vi "Construct String Control Sink.vi"(4 "Error Action":T1=enum."Ignore Error and Close Sink", 5 "Buffer Length(0)":u32, 6 "Clear on Shutdown?(F)":bool, 7 "Str Refnum":refnum<vi>, 8 "Log Filter":refnum<class "ILogFilter.lvclass">, 9 "AutoScroll?(F)":bool, 10 "LogFormat":refnum<class "IStringFormat.lvclass">, 11 "LogLevel":T2) -> (3 "String Control Sink out":refnum<class "String Control Sink.lvclass">)   [LabVIEW 2018, in "MVA Framework.lvlib" / "String Control Sink.lvclass"]
doc: "Create a new String Control Sink. Use the auto scroll flag to enable or disable automatic scrolling of the string indicator. If a custom log format isn't injected, a default string format is used. Use the clear on shutdown flag to clear the string indicator on close. Input a non-zero buffer value to use a rotating, fixed size string buffer."
uses:
  String Control Sink.lvclass
  Composed Log/Log Sink/Log Sink.lvclass
  String Log Sink/String Log Sink.lvclass
  Composed Log/Types/Log Level.ctl
  Composed Log/Composed Log.lvlib
  IStringFormat/IStringFormat.lvclass
  Composed Log/ILogFilter/ILogFilter.lvclass
  Composed Log/Log Sink/Sink Error Actions ENUM.ctl
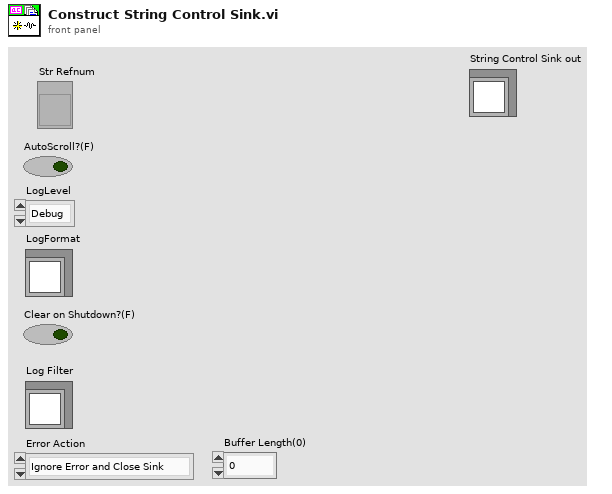
[diagram p1: front panel]
types:
  T1 = typedef "MVA Framework.lvlib/Composed Log.lvlib/Log Sink.lvclass/Sink Error Actions ENUM.ctl" = enum16{"Ignore Error and Continue", "Ignore Error and Close Sink", "Report Error and Close Sink"}
  T2 = typedef "MVA Framework.lvlib/Composed Log.lvlib/Log Level.ctl" = enum16{"Debug", "Info", "Warning", "Error", "Critical"}
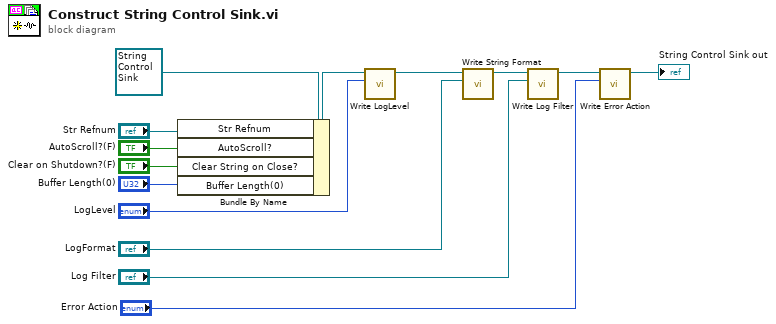
[diagram p0: block diagram]
diagram:
  n1 = Bundle By Name(cluster=refnum<class "String Control Sink.lvclass"> refnum ("String Control Sink in"), "Str Refnum"="Str Refnum", "AutoScroll?"="AutoScroll?(F)", "Clear String on Close?"="Clear on Shutdown?(F)", "Buffer Length(0)"="Buffer Length(0)") -> (w12:refnum<class "String Control Sink.lvclass">)
  n2 = call "Write LogLevel.vi"("LogLevel"="LogLevel", "Log Sink in"=w12) -> ("Log Sink out"=w10:refnum<class "String Control Sink.lvclass">)  [unwired: 8 in, 1 out]
  n3 = call "Write String Format.vi"("StringFormat"="LogFormat", "String Log Sink in"=w10) -> ("String Log Sink out"=w6:refnum<class "String Control Sink.lvclass">)  [unwired: 8 in, 1 out]
  n4 = call "Write Log Filter.vi"("Log Filter"="Log Filter", "Log Sink in"=w6) -> ("Log Sink out"=w4:refnum<class "String Control Sink.lvclass">)  [unwired: 8 in, 1 out]
  n5 = call "Write Error Action.vi"("Error Action"="Error Action", "Log Sink in"=w4) -> ("Log Sink out"=→"String Control Sink out":refnum<class "String Control Sink.lvclass">)  [unwired: 8 in, 1 out]
